vi "DrawElementOnField.vi"(1 "Intensity":dbl=100.0, 2 "PosY":dbl, 3 "PosX":dbl, 4 "Field in":dbl[][](graph)) -> (0 "Field out":dbl[][](graph))   [LabVIEW 2014, in "Field.lvclass"]
uses:
  Field.lvclass
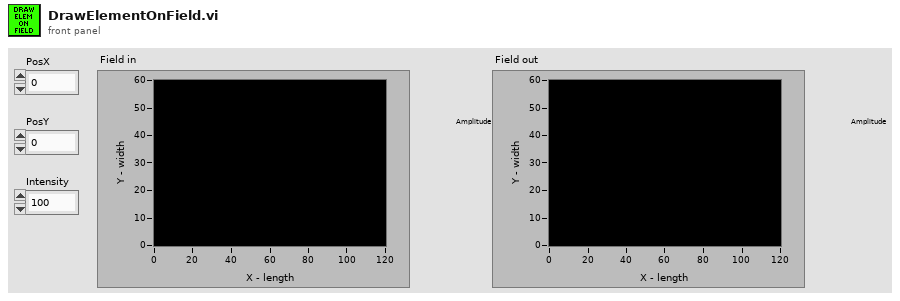
[diagram p1: front panel]
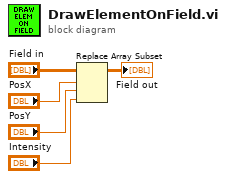
[diagram p0: block diagram]
diagram:
  n1 = Replace Array Subset(array="Field in", new element="Intensity", index (row)="PosX", index (col)="PosY") -> (→"Field out":dbl[][])
